vi "Set Control Value {Variant}__ogtk.vi"(8 "error in (no error)":errorcluster, 9 "Control Name (\"\": use variant name)":string, 10 "Value":variant, 11 "VI Refnum":refnum<vi>) -> (0 "error out":errorcluster, 3 "VI Refnum dup":refnum<vi>)   [LabVIEW 2012]
doc: "Sets the value of the named control to that of the variant data. If <B>Control Name</B> is not specified, then the variant data name of the <B>Value</B> input will be used in its place."
panel:
  # "Please visit http://www.OpenG.org to learn about the\nOpen Source LabVIEW software movement.\n\nNOTICE -- YOU MUST LEAVE THIS NOTICE IN PLACE.  PER THE TERMS OF THE LICENSE BELOW, YOU MAY SUBLICENSE THIS SOFTWARE \nIN ANY WAY THAT DOES NOT CONFLICT WITH THIS LICENSE.\n\n### BSD License (http://www.opensource.org/licenses/bsd-license.php) Begin ###\n \nCopyright (c) 2002, Jean-Pierre Drolet <drolet_jp@hotmail.com>\nCopyright (c) 2002, Jim Kring <jim@jimkring.com>\nCopyright (c) 2011, Jonathon Green <jg@jgcode.net>\n\nAll rights reserved.\n\nRedistribution and use in source and binary forms, with or without modification, are permitted provided that the following conditions are met:\n\n    * Redistributions of source code must retain the above copyright notice, this list of conditions and the following disclaimer.\n    * Redistributions in binary form must reproduce the above copyright notice, this list of conditions and the following disclaimer in the \n       documentation and/or other materials provided with the distribution.\n    * Neither the name of SciWare, James Kring, Inc., nor the names of its contributors may be used to endorse or promote products derived \n       from this software without specific prior written permission.\n\nTHIS SOFTWARE IS PROVIDED BY THE COPYRIGHT HOLDERS AND CONTRIBUTORS \"AS IS\" AND ANY EXPRESS OR IMPLIED WARRANTIES, \nINCLUDING, BUT NOT LIMITED TO, THE IMPLIED WARRANTIES OF MERCHANTABILITY AND FITNESS FOR A PARTICULAR PURPOSE ARE \nDISCLAIMED. IN NO EVENT SHALL THE COPYRIGHT OWNER OR CONTRIBUTORS BE LIABLE FOR ANY DIRECT, INDIRECT, INCIDENTAL,\n SPECIAL, EXEMPLARY, OR CONSEQUENTIAL DAMAGES (INCLUDING, BUT NOT LIMITED TO, PROCUREMENT OF SUBSTITUTE GOODS OR \nSERVICES; LOSS OF USE, DATA, OR PROFITS; OR BUSINESS INTERRUPTION) HOWEVER CAUSED AND ON ANY THEORY OF LIABILITY, \nWHETHER IN CONTRACT, STRICT LIABILITY, OR TORT (INCLUDING NEGLIGENCE OR OTHERWISE) ARISING IN ANY WAY OUT OF THE USE \nOF THIS SOFTWARE, EVEN IF ADVISED OF THE POSSIBILITY OF SUCH DAMAGE.\n\n### BSD License End ###"
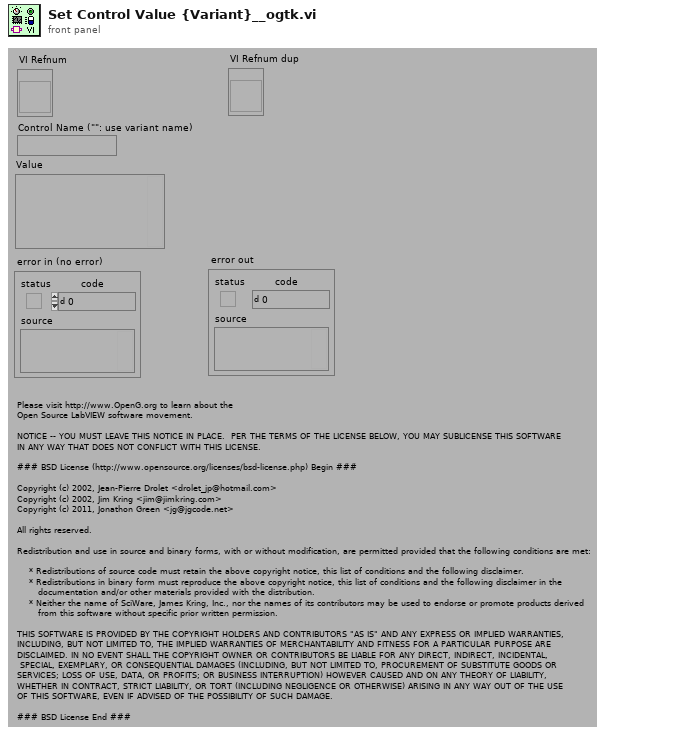
[diagram p1: front panel]
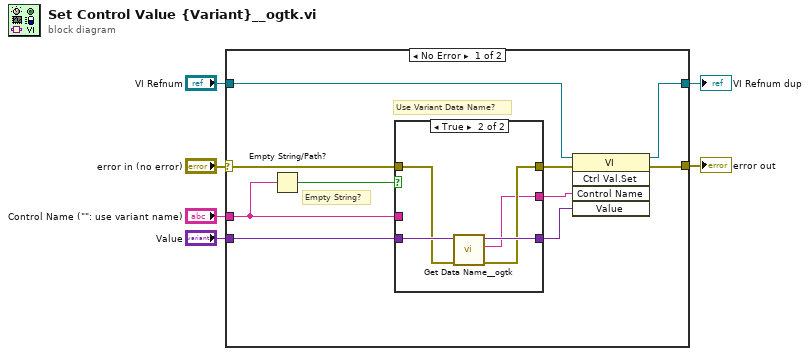
[diagram p0: block diagram]
diagram:
  n1 = case shown="No Error" "error in (no error)" {
    selector: "error in (no error)" -> [w8 w26]
    tunnel: "VI Refnum" -> [w16 w25]
    tunnel: [w15 w25] -> w5
    tunnel: [w14 w26] -> w4
    tunnel: "Value" -> [w13 _]
    tunnel: "Control Name (\"\": use variant name)" -> [w9 _]
    frame No Error {
      # "Use Variant Data Name?"
      # "Empty String?"
      n2 = Empty String/Path?(string/path=w9) -> (empty?=w10:bool)
      n3 = case shown="True" w10 {
        tunnel: w13 -> [w17 w24]
        tunnel: [w17 w23] -> w7
        tunnel: w9 -> [w19 _]
        tunnel: w8 -> [w18 w22]
        tunnel: [w18 w21] -> w12
        tunnel: [w19 w20] -> w11
        frame False {
        }
        frame True {
          n4 = call <userlib>:"Get Data Name__ogtk.vi"("error in (no error)"=w22, "Data"=w24) -> ("error out"=w21:errorcluster, "Data Name"=w20:string, "Data dup"=w23:variant)  [unwired: 7 in]
        }
      }
      n5 = invoke class="VI" method="Ctrl Val.Set"(reference=w16, error in=w12, "Control Name"=w11, "Value"=w7) -> (reference out=w15:refnum<vi>, error out=w14:errorcluster)  [unwired: 1 in, 3 out]
    }
    frame Error {
    }
  }
  "error out" <- w4
  "VI Refnum dup" <- w5
